vi "sub_cal-b_linear.vi"(10 "커서.커서 위치":T1 caption="point", 11 "a":dbl) -> (3 "b":dbl)   [LabVIEW 2019]
uses:
  <vilib>/Utility/miscctls.llb/LVPointDoubleTypeDef.ctl
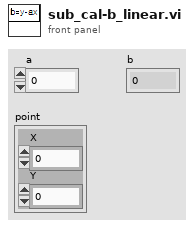
[diagram p1: front panel]
types:
  T1 = typedef "LVPointDoubleTypeDef.ctl" = cluster{"X":dbl, "Y":dbl}
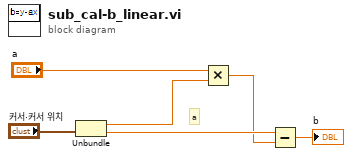
[diagram p0: block diagram]
diagram:
  # "a"
  n1 = Unbundle("커서.커서 위치") -> ("X"=w1:dbl, "Y"=w5:dbl)
  n2 = Multiply(x="a", y=w1) -> (x*y=w4:dbl)
  n3 = Subtract(x=w5, y=w4) -> (x-y=→"b":dbl)
